vi "Ultramat 23 Create Data Array.vi"(7 "AFCO Data":string[][](array[string]), 8 "error in (no error)":errorcluster, 9 "Measured variables":T3[](array[typedef]), 10 "Measurements":cluster{"Measured value":dbl, "Dimension":T4}[](array[cluster]), 11 "Message Header":T1 {"Source Address" format="%.0x"; "Target Address" format="%.0x"}) -> (0 "error out":errorcluster, 3 "Data Array":string[][](array[string]))   [LabVIEW 2023]
uses:
  instr.lib/Siemens ELAN/Unit Dimensions.ctl
  instr.lib/Siemens ELAN/Measured variables.ctl
  instr.lib/Siemens ELAN/Message Header.ctl
  instr.lib/Siemens ELAN/Channel Status.ctl
  instr.lib/Siemens ELAN/Siemens ELAN.lvlib
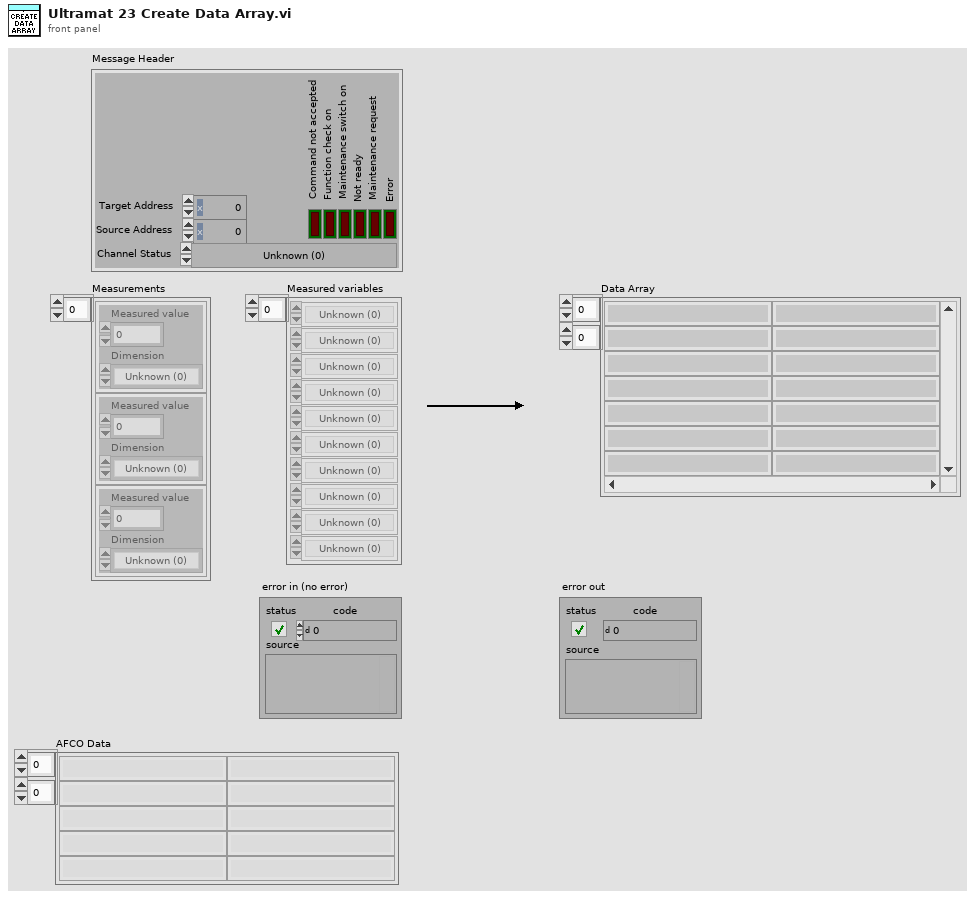
[diagram p1: front panel]
types:
  T1 = typedef "Siemens ELAN.lvlib/Message Header.ctl" = cluster{"Target Address":u8, "Source Address":u8, "Error":bool, "Maintenance request":bool, "Not ready":bool, "Maintenance switch on":bool, "Function check on":bool, "Command not accepted":bool, "Channel Status":T2}
  T2 = typedef "Siemens ELAN.lvlib/Channel Status.ctl" = enum8{"Unknown (0)", "Warm-up", "Pause", "Standby", "Measure", "Zero calibration", "Adjust component slope", "Unknown (7)", "Adjust curve dip", "Adjust linearization sensitivity", "Adjust temperature compensation", "Adjust pressure compensation", "Adjust linearization zero", "Adjust flow sensor", "Autocal", "Adjust phase", "Zero calibration of O2 sensor", "Synchronous zero calibration", "Purging for synchronous zero calibration", "Adjust analog output", "Adjust analog input", "Cleaning", "Unknown (>21)"}
  T3 = typedef "Siemens ELAN.lvlib/Measured variables.ctl" = enum8{"Unknown (0)", "No component", "CO", "CO2", "CH4", "C6H14", "SO2", "NO", "NO2", "CHClF2 (R22)", "C3H8", "C4H10", "O2", "C5H12", "HC", "Pressure", "pH", "Temperature", "C2H4", "C2H2", "C3H6", "C4H6", "C4H8", "C2H6", "NH3", "N2O", "C6H6", "SF6", "CH3OH", "C2H5OH", "CH2Cl2", "C2H4Cl2", "CH3Cl", "C2H4O", "H2O (vapor)", "G/l", "Unknown (36)", "Unknown (37)", "Unknown (38)", "Unknown (39)", "Unknown (40)", "Unknown (41)", "Unknown (42)", "Unknown (43)", "Unknown (44)", "Unknown (45)", "Unknown (46)", "Unknown (47)", "Unknown (48)", "Unknown (49)", "Unknown (50)", "Unknown (51)", "Unknown (52)", "Unknown (53)", "Unknown (54)", "Unknown (55)", "Unknown (56)", "Unknown (57)", "Unknown (58)", "Unknown (59)", "Unknown (60)", "Unknown (61)", "Unknown (62)", "Unknown (63)", "Unknown (64)", "Unknown (65)", "Unknown (66)", "Unknown (67)", "Unknown (68)", "Unknown (69)", "Unknown (70)", "Unknown (71)", "Unknown (72)", "Unknown (73)", "Unknown (74)", "Unknown (75)", "Unknown (76)", "Unknown (77)", "Unknown (78)", "Unknown (79)", "Unknown (80)", "Unknown (81)", "Unknown (82)", "Unknown (83)", "Unknown (84)", "Unknown (85)", "Unknown (86)", "Unknown (87)", "Unknown (88)", "Unknown (89)", "Unknown (90)", "Unknown (91)", "Unknown (92)", "Unknown (93)", "Unknown (94)", "Unknown (95)", "Unknown ((96)", "Unknown (97)", "Unknown (98)", "Unknown (99)", "Ambient Pressure", "Unknown (>100)"}
  T4 = typedef "Siemens ELAN.lvlib/Unit Dimensions.ctl" = enum8{"Unknown (0)", "Pure number", "ppm", "ppb", "vpm", "vpm C1", "vpm C3", "vpm C6", "mg C/m^3", "mg/m^3", "%", "% v/v", "% of range", "% saturation", "%/°C", "%/K", "% w/w", "mV/pH", "mV/mbar", "nA/mbar", "S/m", "S/cm", "mS/m", "mS/cm", "uS/m", "uS/cm", "s", "min", "hr", "pA", "mA", "uV", "mV", "V", "mbar", "hPa", "ml/min", "kohm", "MOhm", "S", "°C", "Hz", "pH", "ug/l", "mg/l", "l/min", "uA", "mg/dm^3", "kPa", "kohm*cm", "MOhm*cm", "°", "Unknown (>51)"}
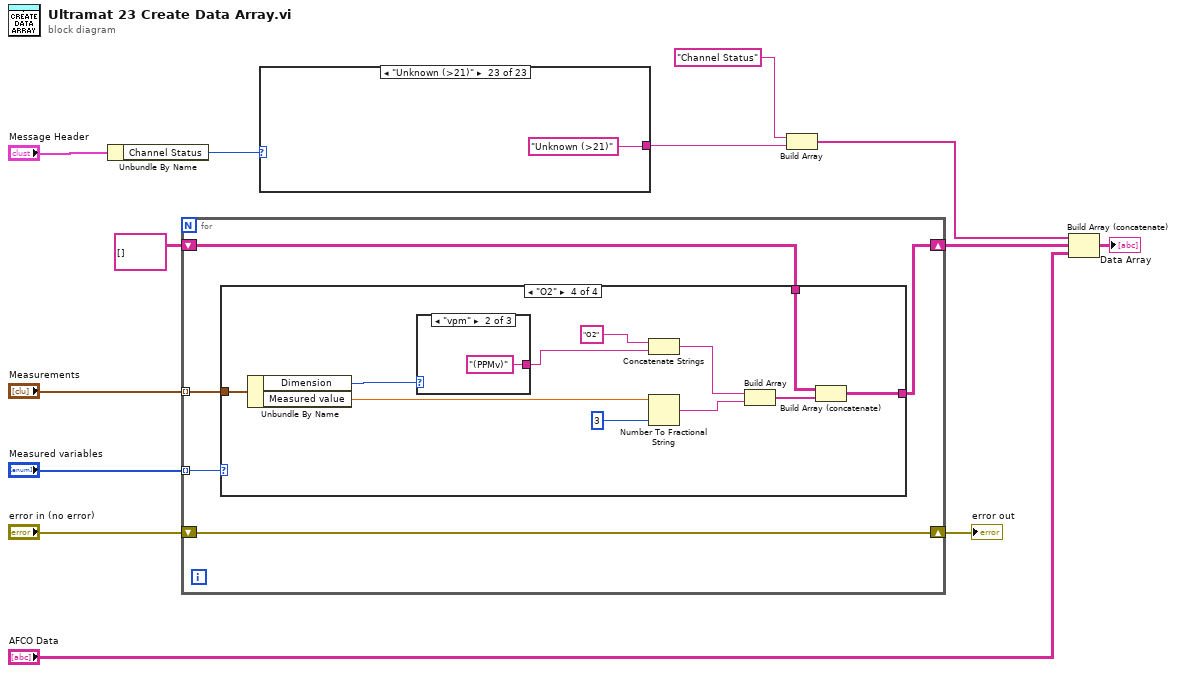
[diagram p0: block diagram]
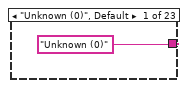
[diagram p2: hidden frame]
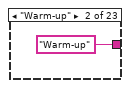
[diagram p3: hidden frame]
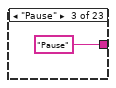
[diagram p4: hidden frame]
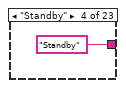
[diagram p5: hidden frame]
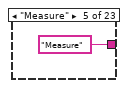
[diagram p6: hidden frame]
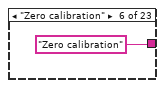
[diagram p7: hidden frame]
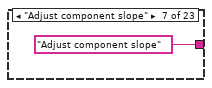
[diagram p8: hidden frame]
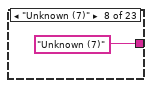
[diagram p9: hidden frame]
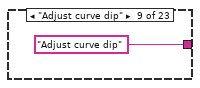
[diagram p10: hidden frame]
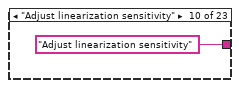
[diagram p11: hidden frame]
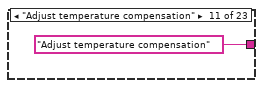
[diagram p12: hidden frame]
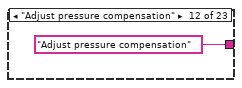
[diagram p13: hidden frame]
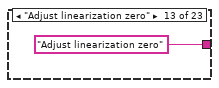
[diagram p14: hidden frame]
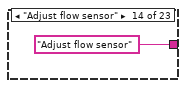
[diagram p15: hidden frame]
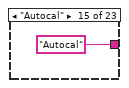
[diagram p16: hidden frame]
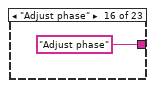
[diagram p17: hidden frame]
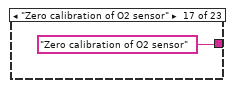
[diagram p18: hidden frame]
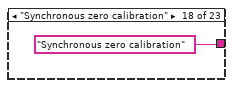
[diagram p19: hidden frame]
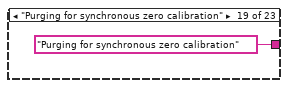
[diagram p20: hidden frame]
diagram:
  n1 = Unbundle By Name("Message Header") -> ("Channel Status"=w7:T2)
  n2 = for {
    tunnel: "Measured variables" -> [w18] mode=indexing
    tunnel: "Measurements" -> [w17] mode=indexing
    shift-right: [w15] -> w4
    shift-left: string[][] [] -> [w16]
    shift-right: [w14] -> w9
    shift-left: "error in (no error)" -> [w14]
    n3 = case shown="\"O2\"" w18 {
      tunnel: w17 -> [_ w30 w38 w52]
      tunnel: w16 -> [w19 w22 w36 w50]
      tunnel: [w19 w21 w35 w49] -> w15
      frame "Unknown (0)", Default {
      }
      frame "CO" {
        n4 = Unbundle By Name(w30) -> ("Dimension"=w20:T4, "Measured value"=w27:dbl)
        n5 = case shown="\"vpm\"" w20 {
          tunnel: ["(Unknown)" "(PPMv)" "(%)"] -> w28
          frame "Unknown (0)", Default {
          }
          frame "vpm" {
          }
          frame "%" {
          }
        }
        n6 = Concatenate Strings("CO", w28) -> (w25:string)
        n7 = Number To Fractional String(number=w27, precision (6)=i16 3) -> (F-format string=w24:string)  [unwired: 2 in]
        n8 = Build Array(w25, w24) -> (w23:string[])
        n9 = Build Array (concatenate)(w22, w23) -> (w21:string[][])
      }
      frame "CO2" {
        n10 = Unbundle By Name(w38) -> ("Dimension"=w34:T4, "Measured value"=w43:dbl)
        n11 = case shown="\"%\"" w34 {
          tunnel: ["(Unknown)" "(PPMv)" "(%)"] -> w44
          frame "Unknown (0)", Default {
          }
          frame "vpm" {
          }
          frame "%" {
          }
        }
        n12 = Concatenate Strings("CO2", w44) -> (w42:string)
        n13 = Number To Fractional String(number=w43, precision (6)=i16 3) -> (F-format string=w41:string)  [unwired: 2 in]
        n14 = Build Array(w42, w41) -> (w37:string[])
        n15 = Build Array (concatenate)(w36, w37) -> (w35:string[][])
      }
      frame "O2" {
        n16 = Unbundle By Name(w52) -> ("Dimension"=w48:T4, "Measured value"=w57:dbl)
        n17 = case shown="\"vpm\"" w48 {
          tunnel: ["(Unknown)" "(PPMv)" "(%)"] -> w58
          frame "Unknown (0)", Default {
          }
          frame "vpm" {
          }
          frame "%" {
          }
        }
        n18 = Concatenate Strings("O2", w58) -> (w56:string)
        n19 = Number To Fractional String(number=w57, precision (6)=i16 3) -> (F-format string=w55:string)  [unwired: 2 in]
        n20 = Build Array(w56, w55) -> (w51:string[])
        n21 = Build Array (concatenate)(w50, w51) -> (w49:string[][])
      }
    }
  }
  "error out" <- w9
  n22 = case shown="\"Unknown (>21)\"" w7 {
    tunnel: ["Unknown (0)" "Warm-up" "Pause" "Standby" "Measure" "Zero calibration" "Adjust component slope" "Unknown (7)" "Adjust curve dip" "Adjust linearization sensitivity" "Adjust temperature compensation" "Adjust pressure compensation" "Adjust linearization zero" "Adjust flow sensor" "Autocal" "Adjust phase" "Zero calibration of O2 sensor" "Synchronous zero calibration" "Purging for synchronous zero calibration" "Adjust analog output" "Adjust analog input" "Cleaning" "Unknown (>21)"] -> w5
    frame "Unknown (0)", Default {
    }
    frame "Warm-up" {
    }
    frame "Pause" {
    }
    frame "Standby" {
    }
    frame "Measure" {
    }
    frame "Zero calibration" {
    }
    frame "Adjust component slope" {
    }
    frame "Unknown (7)" {
    }
    frame "Adjust curve dip" {
    }
    frame "Adjust linearization sensitivity" {
    }
    frame "Adjust temperature compensation" {
    }
    frame "Adjust pressure compensation" {
    }
    frame "Adjust linearization zero" {
    }
    frame "Adjust flow sensor" {
    }
    frame "Autocal" {
    }
    frame "Adjust phase" {
    }
    frame "Zero calibration of O2 sensor" {
    }
    frame "Synchronous zero calibration" {
    }
    frame "Purging for synchronous zero calibration" {
    }
    frame "Adjust analog output" {
    }
    frame "Adjust analog input" {
    }
    frame "Cleaning" {
    }
    frame "Unknown (>21)" {
    }
  }
  n23 = Build Array("Channel Status", w5) -> (w3:string[])
  n24 = Build Array (concatenate)(w3, w4, "AFCO Data") -> (→"Data Array":string[][])
